vi "mqtt_broker.vi"() -> ()   [LabVIEW 2024]
uses:
  <vilib>/LabVIEW Open Source Project/Connection/Connection.TCP/Connection.TCP.lvclass
  C:/Program Files (x86)/National Instruments/LabVIEW 2024/vi.lib/LabVIEW Open Source Project/Connection/Connection/Connection.lvclass
  <vilib>/G Open Source Project for LabVIEW/MQTT Broker/Server class/Server.lvclass
  C:/Program Files (x86)/National Instruments/LabVIEW 2024/vi.lib/LabVIEW Open Source Project/MQTT Connection/MQTT_Base/Base Class/MQTT_Base.lvclass
  <vilib>/LabVIEW Open Source Project/MQTT Connection/MQTT_Base/Base Class/MQTT_Base.lvclass
panel:
  out "Nb Connections":u32
  in  "stop":bool
  out "error server":errorcluster
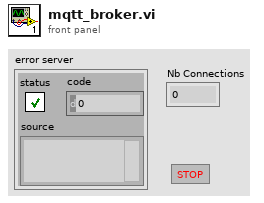
[diagram p1: front panel]
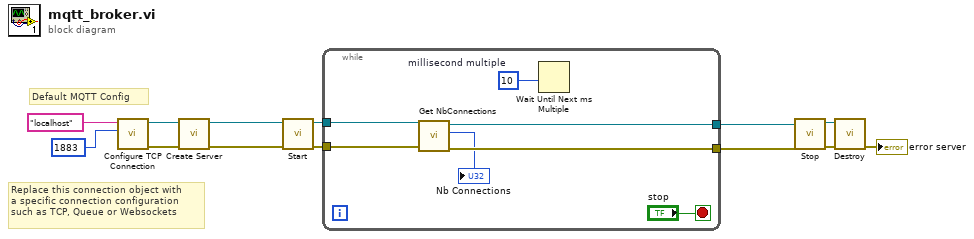
[diagram p0: block diagram]
diagram:
  # "Default MQTT Config"
  # "Replace this connection object with\na specific connection configuration\nsuch as TCP, Queue or Websockets"
  n1 = call <vilib>:"Configure TCP Connection.vi"("remote port (80)"=u16 1883, "address (localhost)"="localhost") -> ("error out"=w7:errorcluster, "Connection.TCP"=w13:refnum<class "Connection.TCP.lvclass">)  [unwired: 8 in]
  n2 = call <vilib>:"Create Server.vi"("error in (no error)"=w7, "Connection Configuration"=w13) -> ("error out"=w5:errorcluster, "Server"=w6:refnum<class "Server.lvclass">)  [unwired: 8 in]
  n3 = call <vilib>:"Start.vi"("error in (no error)"=w5, "MQTT_Base in"=w6) -> ("error out"=w3:errorcluster, "MQTT_Base out"=w4:refnum<class "Server.lvclass">)  [unwired: 7 in, 1 out]
  n4 = while {
    tunnel: w4 -> [w20]
    tunnel: w3 -> [w19]
    tunnel: [w16] -> w2
    tunnel: [w15] -> w1
    stop <- "stop" stop-if-true
    w17 = u32 10  # millisecond multiple
    n5 = call <vilib>:"Get NbConnections.vi"("error in (no error)"=w19, "Server in"=w20) -> ("error out"=w15:errorcluster, "Nb Connections"=→"Nb Connections":u32, "Server out"=w16:refnum<class "Server.lvclass">)  [unwired: 7 in]
    n6 = Wait Until Next ms Multiple(millisecond multiple=w17) -> ()  [unwired: 1 out]
  }
  n7 = call <vilib>:"Stop.vi"("error in (no error)"=w1, "MQTT_Base in"=w2) -> ("error out"=w12:errorcluster, "MQTT_Base out"=w11:refnum<class "Server.lvclass">)  [unwired: 7 in, 1 out]
  n8 = call <vilib>:"Destroy.vi"("error in (no error)"=w12, "MQTT_Base in"=w11) -> ("error out"=→"error server":errorcluster)  [unwired: 8 in, 1 out]
